vi "4Pi OIA -Test NCC Shift Amount.vi"() -> ()   [LabVIEW 2016]
uses:
  Tools/2D Gaussian Fit/2D Gaussian - Type Defs/2D Gaussian - Best Fit Parameters.ctl
panel:
  out "Fit Shift Amount (px)":dbl[](array[numeric])
  out "NCC Shift Amount (px)":dbl[](array[numeric])
  out "NCC Fit Result":T1
  out "NCC Image":dbl[][](graph)
  out "Image 02":u16[][](graph)
  in  "Image 02 Parameters":dbl[](array[numeric])
  out "Image 01":u16[][](graph)
  in  "Columns (X)":i32
  in  "Rows (Y)":i32
  in  "Image 01 Parameters":dbl[](array[numeric])
  # "Upper Obj"
  # "Lower Obj"
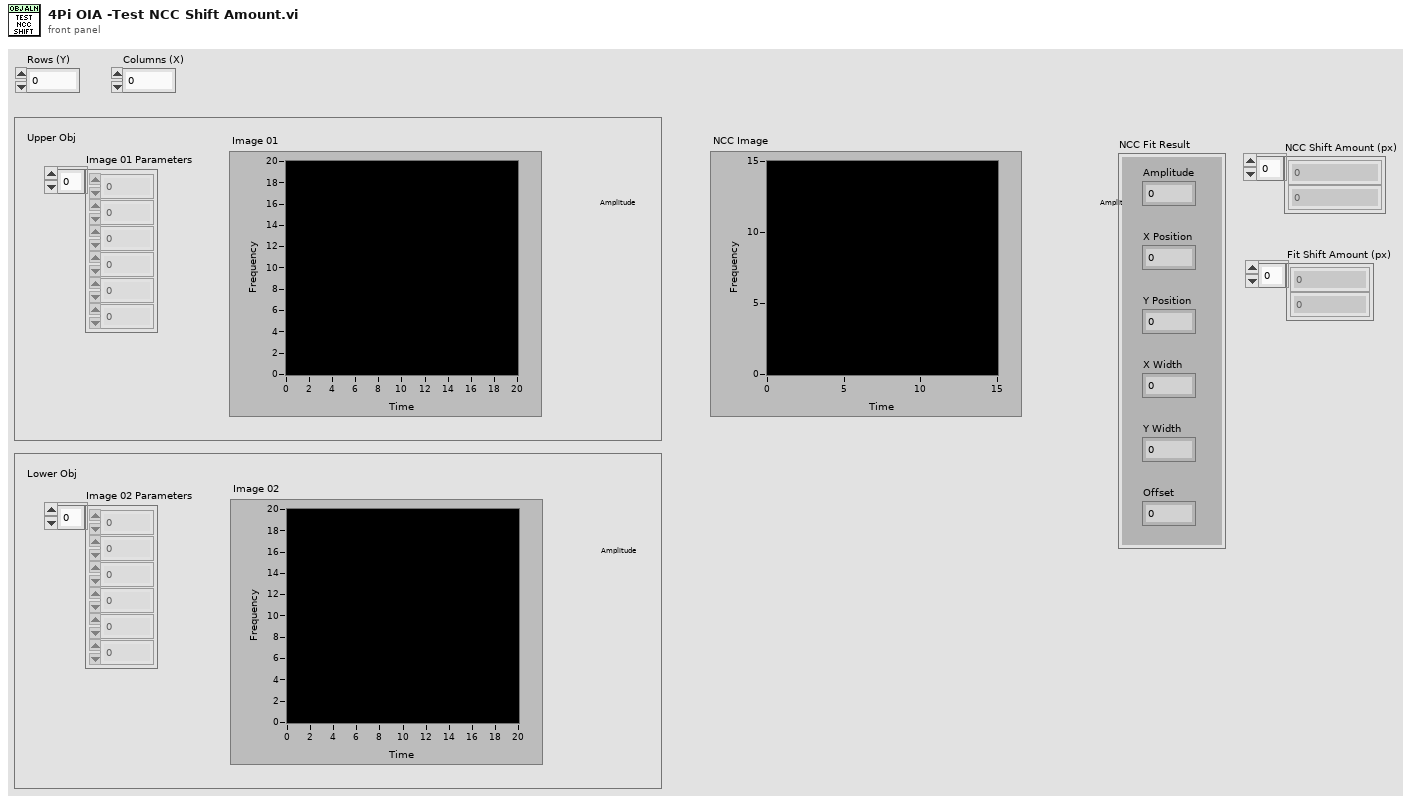
[diagram p1: front panel]
types:
  T1 = typedef "2D Gaussian - Best Fit Parameters.ctl" = cluster{"Amplitude":dbl, "X Position":dbl, "Y Position":dbl, "X Width":dbl, "Y Width":dbl, "Offset":dbl}
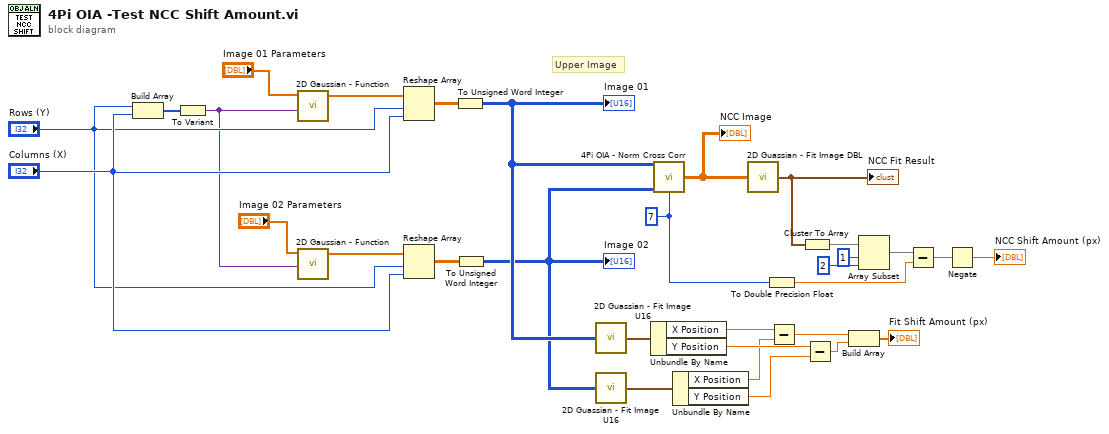
[diagram p0: block diagram]
diagram:
  w15 = 7 ("Half Shift")
  # "Upper Image"
  n1 = Build Array("Rows (Y)", "Columns (X)") -> (w29:i32[])
  n2 = To Variant(anything=w29) -> (Variant=w24:variant)
  n3 = call "2D Gaussian - Function.vi"("data"=w24, "a"="Image 01 Parameters") -> ("f(X,a)"=w30:dbl[])  [unwired: 2 in, 2 out]
  n4 = call "2D Gaussian - Function.vi"("data"=w24, "a"="Image 02 Parameters") -> ("f(X,a)"=w27:dbl[])  [unwired: 2 in, 2 out]
  n5 = Reshape Array(w30, "Rows (Y)", "Columns (X)") -> (w28:dbl[][])
  n6 = Reshape Array(w27, "Rows (Y)", "Columns (X)") -> (w22:dbl[][])
  n7 = To Unsigned Word Integer(number=w28) -> (unsigned 16bit integer=w4:u16[][])
  "Image 01" <- w4
  n8 = To Unsigned Word Integer(number=w22) -> (unsigned 16bit integer=w3:u16[][])
  "Image 02" <- w3
  n9 = call "2D Guassian - Fit Image U16.vi"("Image In (U16)"=w4) -> ("Best Fit Params"=w5:T1)  [unwired: 14 in]
  n10 = call "2D Guassian - Fit Image U16.vi"("Image In (U16)"=w3) -> ("Best Fit Params"=w12:T1)  [unwired: 14 in]
  n11 = Unbundle By Name(w5) -> ("X Position"=w11:dbl, "Y Position"=w10:dbl)
  n12 = call "4Pi OIA - Norm Cross Corr.vi"("Image 01"=w4, "Image 02"=w3, "Half Shift"=w15) -> ("Norm Cross Corr Result"=w21:dbl[][])  [unwired: 12 in]
  "NCC Image" <- w21
  n13 = Unbundle By Name(w12) -> ("X Position"=w9:dbl, "Y Position"=w8:dbl)
  n14 = call "2D Guassian - Fit Image DBL.vi"("Image In (DBL)"=w21) -> ("Best Fit Params"=w20:T1)  [unwired: 14 in]
  "NCC Fit Result" <- w20
  n15 = To Double Precision Float(number=w15) -> (double precision float=w14:dbl)
  n16 = Subtract(x=w11, y=w9) -> (x-y=w7:dbl)
  n17 = Cluster To Array(cluster=w20) -> (array=w19:dbl[])
  n18 = Subtract(x=w10, y=w8) -> (x-y=w6:dbl)
  n19 = Build Array(w7, w6) -> (→"Fit Shift Amount (px)":dbl[])
  n20 = Array Subset(array=w19, index=1, length=2 ("index")) -> (w16:dbl[])
  n21 = Subtract(x=w16, y=w14) -> (x-y=w13:dbl[])
  n22 = Negate(x=w13) -> (-x=→"NCC Shift Amount (px)":dbl[])
